vi "CalcLineAccuracy.vi"(11 "MainData":T1) -> (3 "Good ?":bool)   [LabVIEW 2020]
uses:
  typeDef/MainDataCluster.ctl
  <vilib>/picture/picture.llb/imagedata.ctl
  typeDef/StateMachineEnum.ctl
  typeDef/EventData.ctl
  typeDef/EndType.ctl
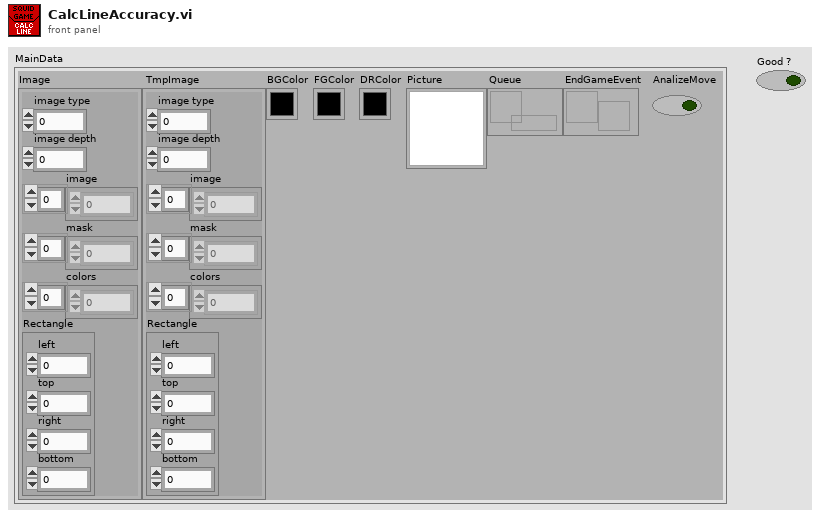
[diagram p1: front panel]
types:
  T1 = typedef "MainDataCluster.ctl" = cluster{"Image":T2, " TmpImage":T2, "BGColor":u32, "FGColor":u32, "DRColor":u32, "Picture":picture, "Queue ":refnum<queue>, "EndGameEvent":refnum<user-event>, "AnalizeMove":bool}
  T2 = typedef "imagedata.ctl" = cluster{"image type":i32, "image depth":i32, "image":u8[], "mask":u8[], "colors":u32[], "Rectangle":cluster{"left":i16, "top":i16, "right":i16, "bottom":i16}}
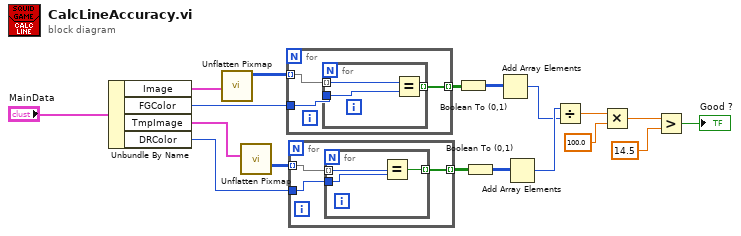
[diagram p0: block diagram]
diagram:
  n1 = Unbundle By Name("MainData") -> ("Image"=w13:T2, "FGColor"=w14:u32, "TmpImage"=w15:T2, "DRColor"=w16:u32)
  n2 = call <vilib>:"Unflatten Pixmap.vi"("image data"=w13) -> ("24-bit pixmap"=w1:u32[][])  [unwired: 4 in, 6 out]
  n3 = call <vilib>:"Unflatten Pixmap.vi"("image data"=w15) -> ("24-bit pixmap"=w10:u32[][])  [unwired: 4 in, 6 out]
  n4 = for {
    tunnel: [w21] -> w8 mode=indexing
    tunnel: w14 -> [w20]
    tunnel: w1 -> [w19] mode=indexing
    n5 = for {
      tunnel: [w24] -> w21 mode=indexing
      tunnel: w20 -> [w23]
      tunnel: w19 -> [w22] mode=indexing
      n6 = Equal?(x=w22, y=w23) -> (x = y?=w24:bool)
    }
  }
  n7 = for {
    tunnel: w10 -> [w27] mode=indexing
    tunnel: [w26] -> w12 mode=indexing
    tunnel: w16 -> [w25]
    n8 = for {
      tunnel: w27 -> [w30] mode=indexing
      tunnel: [w29] -> w26 mode=indexing
      tunnel: w25 -> [w28]
      n9 = Equal?(x=w30, y=w28) -> (x = y?=w29:bool)
    }
  }
  n10 = Boolean To (0,1)(Boolean=w8) -> (0, 1=w9:i16[][])
  n11 = Boolean To (0,1)(Boolean=w12) -> (0, 1=w11:i16[][])
  n12 = Add Array Elements(numeric array=w9) -> (sum=w6:i16)
  n13 = Add Array Elements(numeric array=w11) -> (sum=w7:i16)
  n14 = Divide(x=w7, y=w6) -> (x/y=w5:dbl)
  n15 = Multiply(x=w5, y=100.0) -> (x*y=w3:dbl)
  n16 = Greater?(x=w3, y=14.5) -> (0:→"Good ?":bool)
